vi "Catch Nested Value Update.vi"(8 "error in (no error)":errorcluster, 10 "Nested Value Update Msg":refnum<class "Nested Value Update Msg.lvclass">, 11 "ObservingViewModel In":refnum<class "ObservingViewModel.lvclass">) -> (0 "error out":errorcluster, 3 "ObservingViewModel Out":refnum<class "ObservingViewModel.lvclass">)   [LabVIEW 2015, in "ObservingViewModel.lvclass"]
doc: "<License>\nCopyright © 2017 Composed Systems, LLC | All rights reserved\nwww.composed.io\n\nAuthor: Ethan Stern <ethan.stern@composed.io>\n\nThis software is provided \"AS IS\" WITHOUT WARRANTIES, either express or implied, AND IS FOR EDUCATIONAL PURPOSES ONLY.\n</License>"
uses:
  ObservingViewModel.lvclass
  Framework/IViewable/IViewable Messages/Catch Nested Value Change Msg/Nested Value Update Msg.lvclass
  Framework/IViewable/IViewable Messages/Catch Nested Value Change Msg/Nested Value Update Msg.lvclass/Nested Value Update Msg.ctl
  Framework/IViewModel/IViewModel/IViewModel.lvclass/IViewModel.ctl
  Framework/IMediator/IMediator Messages/Publish Msg/Publish Msg.lvclass/Publish Msg.ctl
  <vilib>/ActorFramework/Message Enqueuer/Message Enqueuer.lvclass/Message Enqueuer.ctl
  Framework/IViewable/IViewable Messages/Catch Nested Value Change Msg/Accessors/Read Datum Name.vi
  Framework/IViewable/IViewable Messages/Catch Nested Value Change Msg/Accessors/Read Value.vi
  Framework/IMediator/IMediator Messages/Publish Msg/Send Direct Publish.vi
  <vilib>/ActorFramework/Message Enqueuer/Enqueue.vi
  <vilib>/ActorFramework/Message Priority Queue/Priority Enqueue.vi
  Framework/IMediator/IMediator Messages/Publish Msg/Publish Msg.lvclass
  Framework/IViewModel/IViewModel/IViewModel.lvclass
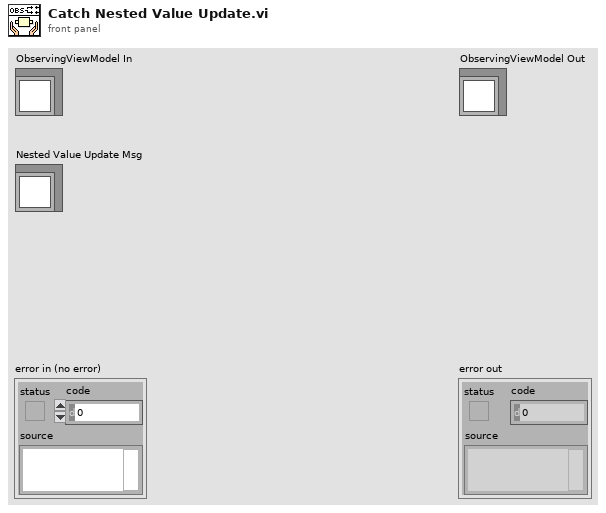
[diagram p1: front panel]
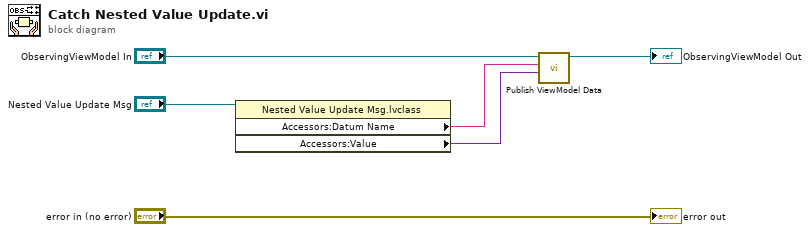
[diagram p0: block diagram]
diagram:
  n1 = property class="Nested Value Update Msg.lvclass"(reference="Nested Value Update Msg") -> ("Accessors:Datum Name"=w2:string, "Accessors:Value"=w1:variant)  [unwired: 1 in, 2 out]
  n2 = call "Publish ViewModel Data.vi"("Data to Publish"=w1, "Datum Name"=w2, "IViewModel In"="ObservingViewModel In") -> ("IViewModel Out"=→"ObservingViewModel Out":refnum<class "ObservingViewModel.lvclass">)  [unwired: 7 in, 1 out]
  "error out" <- "error in (no error)"
